vi "initialize redirection.vi"(11 "Oauth2.LinkedIn":refnum<class "Oauth2.LinkedIn.lvclass">) -> (1 "error out":errorcluster, 3 "Redirect URI":string="http://localhost:58888/Oauth2/Redirect")   [LabVIEW 2017, in "Oauth2.LinkedIn.lvclass"]
uses:
  Oauth2.LinkedIn.lvclass
  Oauth2/Oauth2.lvclass
  <vilib>/LabVIEW Open Source Project/OpenURI/uri/URI.lvclass
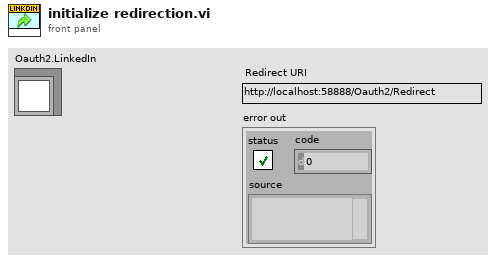
[diagram p1: front panel]
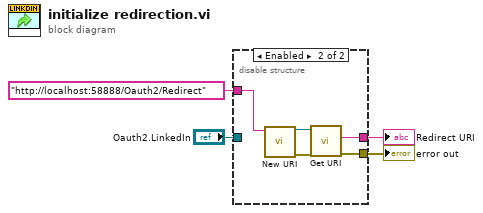
[diagram p0: block diagram]
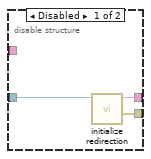
[diagram p2: hidden frame]
diagram:
  n1 = disable-structure shown="Enabled" {
    disable-tunnel: [w7 w9] -> w4
    disable-tunnel: [w6 w10] -> w3
    disable-tunnel: "Oauth2.LinkedIn" -> [w5 _]
    disable-tunnel: "http://localhost:58888/Oauth2/Redirect" ("URI") -> [_ w11]
    frame Disabled {
      n2 = call-parent "initialize redirection.vi"("Oauth2"=w5) -> ("error out"=w7:errorcluster, "Redirect URI"=w6:string)  [unwired: 9 in]
    }
    frame Enabled {
      n3 = call <vilib>:"New URI.vi"("URI"=w11) -> ("error out"=w8:errorcluster, "URI"=w12:refnum<class "URI.lvclass">)  [unwired: 9 in]
      n4 = call <vilib>:"Get URI.vi"("error in (no error)"=w8, "URI in"=w12) -> ("error out"=w9:errorcluster, "URI String"=w10:string)  [unwired: 7 in, 1 out]
    }
  }
  "Redirect URI" <- w3
  "error out" <- w4
